vi "Set Step Name.vi"(8 "error in (no error)":errorcluster, 10 "Standard":string, 11 "Servo to Compression in":refnum<class "Servo to Compression.lvclass">) -> (0 "error out":errorcluster, 2 "Default Step":string, 3 "Servo to Compression out":refnum<class "Servo to Compression.lvclass">)   [LabVIEW 2018, in "Servo to Compression.lvlib" / "Servo to Compression.lvclass"]
uses:
  Servo to Compression.lvclass
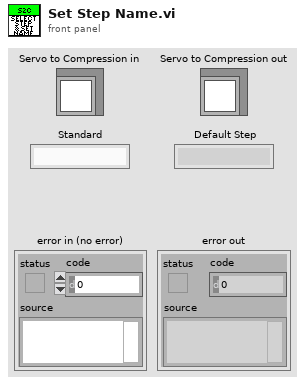
[diagram p1: front panel]
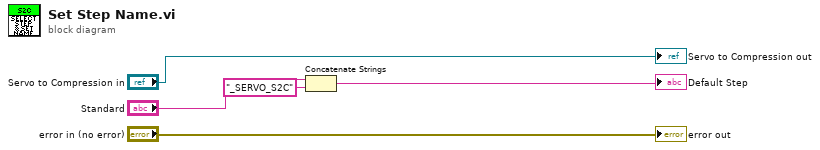
[diagram p0: block diagram]
diagram:
  n1 = Concatenate Strings("Standard", "_SERVO_S2C" ("string")) -> (→"Default Step":string)
  "error out" <- "error in (no error)"
  "Servo to Compression out" <- "Servo to Compression in"
